vi "controlespejo.vi"(10 "cadena entrada":string) -> (1 "x":dbl, 2 "y":dbl)   [LabVIEW 2016]
doc: "Este subVI recibe los datos de la posición del spot en una cadena, los convierte a número flotante y los envia al ni cRIO para poder mover los espejos.\n\nComo entradas están:\n\nLa cadena que contiene los valors de voltaje para mover los espejos.\n\nComo salidas están los valores en x y y de los voltajes aplicados a los espejos."
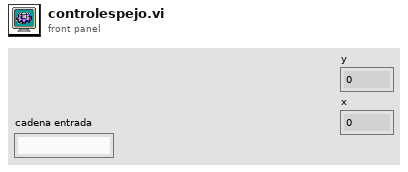
[diagram p1: front panel]
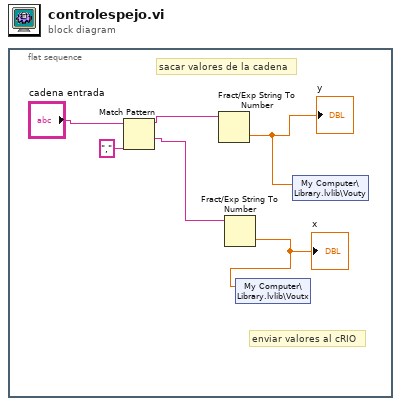
[diagram p0: block diagram]
diagram:
  n1 = flat-sequence {
    frame #0 {
      # "enviar valores al cRIO"
      # "sacar valores de la cadena"
      n2 = Match Pattern(string="cadena entrada", regular expression=",") -> (before substring=w4:string, after substring=w3:string)  [unwired: 1 in, 2 out]
      n3 = Fract/Exp String To Number(string=w4) -> (number=w2:dbl)  [unwired: 3 in, 1 out]
      "y" <- w2
      n4 = Fract/Exp String To Number(string=w3) -> (number=w1:dbl)  [unwired: 3 in, 1 out]
      "x" <- w1
      n5 = shared-variable "My Computer\\Library.lvlib\\Voutx"(w1) -> ()  [unwired: 1 in, 1 out]
      n6 = shared-variable "My Computer\\Library.lvlib\\Vouty"(w2) -> ()  [unwired: 1 in, 1 out]
    }
  }
